vi "checkout.vi"(0 "HGF_ThreadPool_Reference":refnum<class "HGF_Reference.lvclass">, 3 "timeout in ms (-1)":i32=-1, 5 "error in (no error)":errorcluster) -> (14 "dup HGF_ThreadPool_Reference":refnum<class "HGF_Reference.lvclass">, 16 "HGF_ThreadPool":refnum<class "HGF_ThreadPool.lvclass">, 17 "got object?":bool, 19 "error out":errorcluster)   [LabVIEW 2014, in "HGF_BaseClasses.lvlib" / "HGF_ThreadPool.lvclass"]
doc: "Check out the referenced Object.\n\n<B>Attention:</B> Error in is ignored, but forwarded.\nDo not forget to check in again, if you have got the object."
uses:
  HGF_ThreadPool.lvclass
  HGF_Reference/HGF_Reference.lvclass
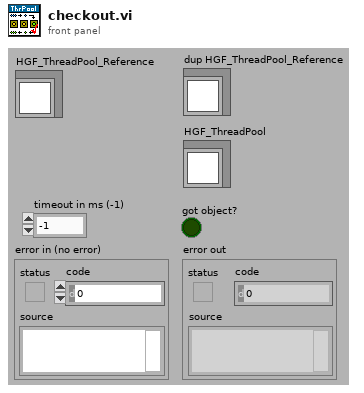
[diagram p1: front panel]
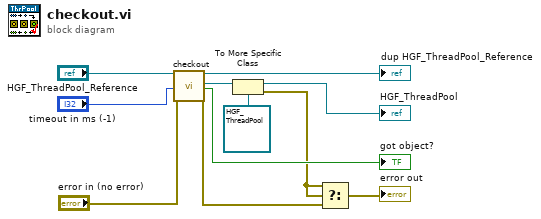
[diagram p0: block diagram]
diagram:
  n1 = call "checkout.vi"("HGF_Reference"="HGF_ThreadPool_Reference", "timeout in ms (-1)"="timeout in ms (-1)", "error in (no error)"="error in (no error)") -> ("dup HGF_Reference"=→"dup HGF_ThreadPool_Reference":refnum<class "HGF_Reference.lvclass">, "Object"=w6:refnum<class>, "got object?"=→"got object?":bool, "error out"=w2:errorcluster)  [unwired: 13 out]
  n2 = To More Specific Class(target class=refnum<class "HGF_ThreadPool.lvclass"> refnum ("HGF_ThreadPool"), reference=w6) -> (specific class reference=→"HGF_ThreadPool":refnum<class "HGF_ThreadPool.lvclass">, error out=w3:errorcluster)  [unwired: 1 in]
  n3 = Select(t=w3, s=w3, f=w2) -> (s? t:f=→"error out":errorcluster)
